vi "MW_Display_Python_Snapshot.vi"(0 "session in":refnum<k35>, 5 "module path":path=path "D:/dev/Guy_Storage/Work/Cancun/MW_Display_Test/Magewell Capture/Capture_LV.py", 11 "error in":errorcluster) -> (4 "session out":refnum<k35>, 6 "module path out":path, 15 "error out":errorcluster)   [LabVIEW 2023]
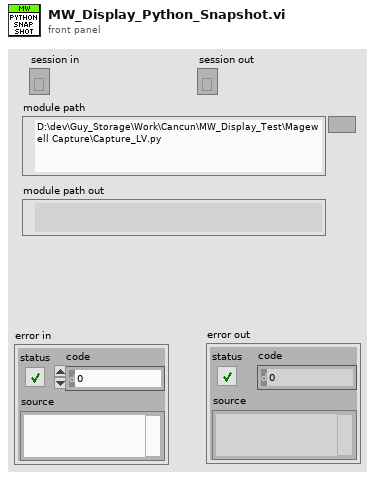
[diagram p1: front panel]
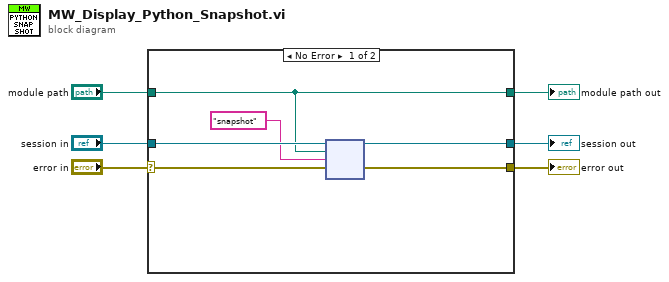
[diagram p0: block diagram]
diagram:
  n1 = case shown="No Error" "error in" {
    selector: "error in" -> [w9 w14]
    tunnel: "module path" -> [w7 w13]
    tunnel: "session in" -> [w12 w15]
    tunnel: [w11 w14] -> w2
    tunnel: [w10 w15] -> w4
    tunnel: [w7 w13] -> w1
    frame No Error {
      n2 = node(w12, w7, "snapshot" ("function name"), w9) -> (w10:refnum<k35>, w11:errorcluster)  [unwired: 2 in, 2 out]
    }
    frame Error {
    }
  }
  "session out" <- w4
  "error out" <- w2
  "module path out" <- w1
